vi "子VI-图像预处理.vi"(7 "图像分辨率":T2, 8 "穿透图":T1(plugin-control), 9 "穿透图原始路径":path) -> (1 "穿透图out":T1(plugin-control))   [LabVIEW 2018]
uses:
  <vilib>/vision/NI_Vision_Development_Module.lvlib
panel:
  in  "stop":bool caption="停止"
  in  "图像预处理":bool
  in  "自定义色彩":bool
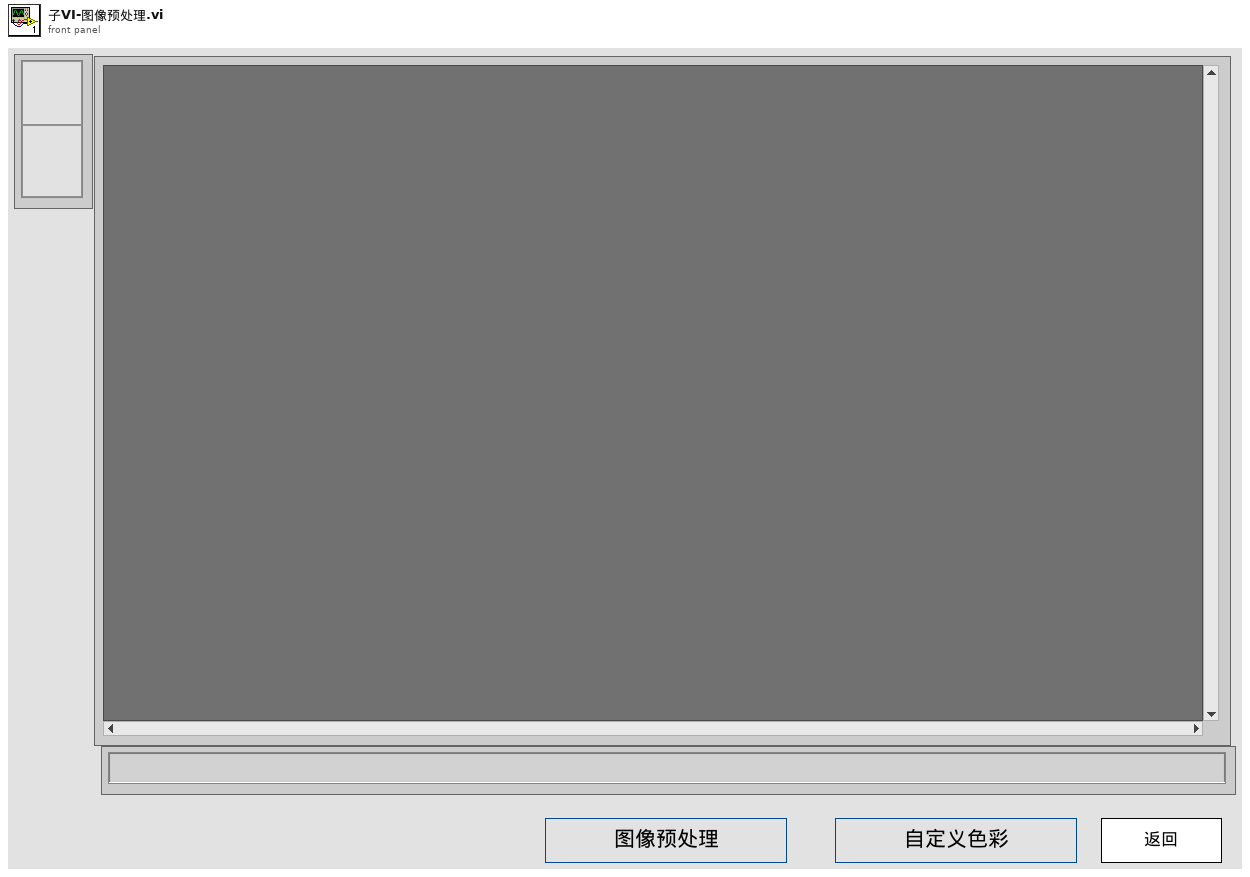
[diagram p1: front panel]
types:
  T1 = typedef "IMAQ Image.ctl" = refnum<image>
  T2 = cluster{"图像X向分辨率（mm/像素）":dbl, "图像Y向分辨率（mm/像素）":dbl}
  T3 = cluster{"Zoom Tool":bool, "Selection Tool":bool, "Pan Tool":bool, "Point Tool":bool, "Line Tool":bool, "Rectangle Tool":bool, "Rotated Rectangle Tool":bool, "Polyline Tool":bool, "Polygon Tool":bool, "Freehand Tool":bool, "Closed Freehand Tool":bool, "Ellipse Tool":bool, "Annulus Tool":bool}
  T4 = enum32{"Linear", "Log", "Exp", "Square", "Square root", "Power X", "Power 1/X"}
  T5 = enum32{"Gray", "Binary", "Gradient", "Rainbow", "Temperature"}
  T6 = enum32{"Invalid", "Standard", "Closed", "Hidden", "Minimized", "Maximized"}
  T7 = typedef "Image Type" = u32
  T8 = cluster{"Red (or Hue) value":u8, "Green (or Sat) value":u8, "Blue (or Light or Val) value":u8}[]
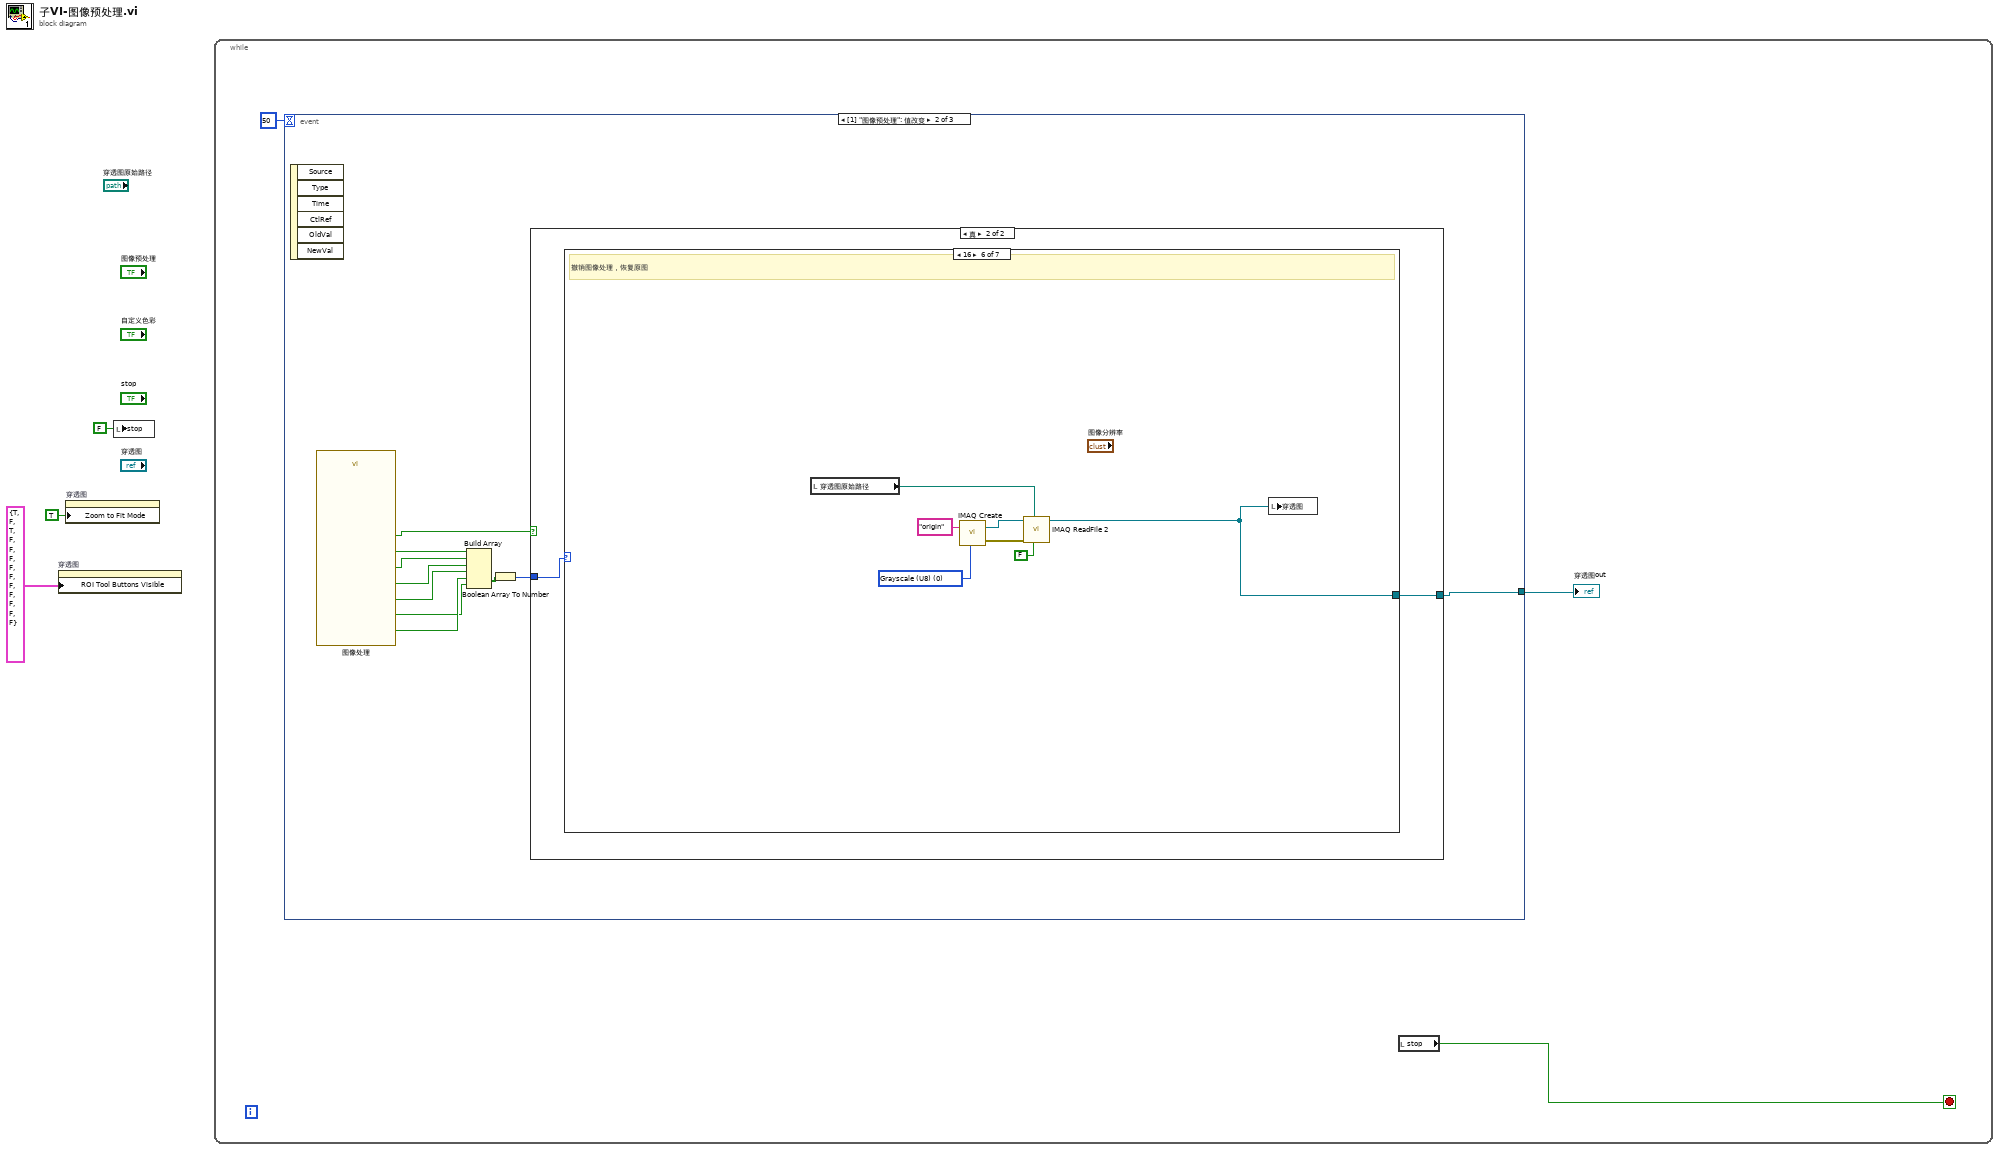
[diagram p0: block diagram]
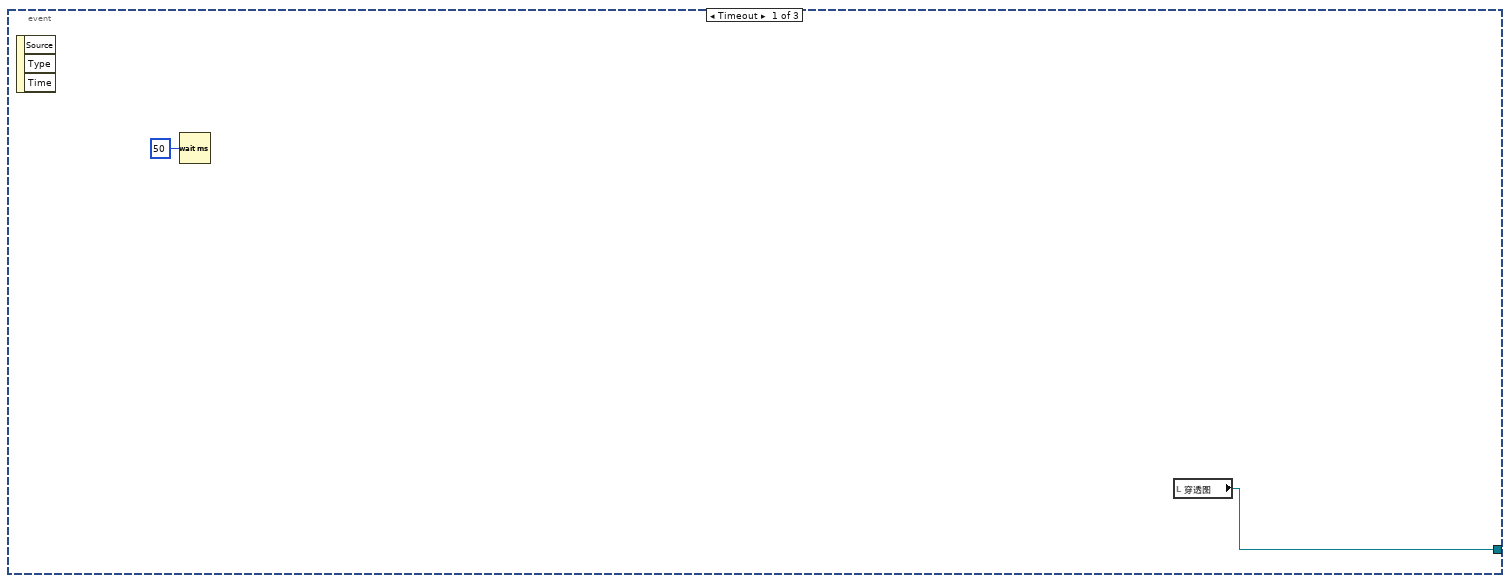
[diagram p2: hidden frame]
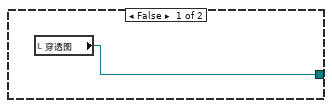
[diagram p3: hidden frame]
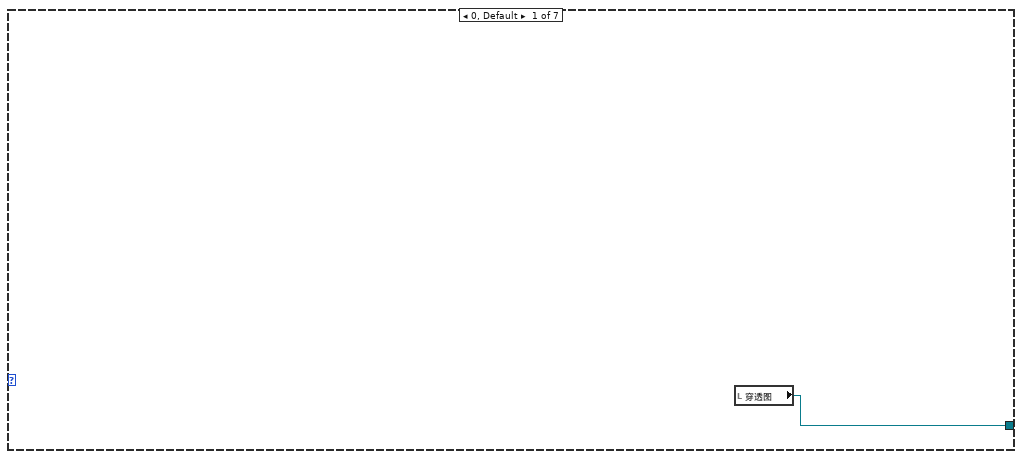
[diagram p4: hidden frame]
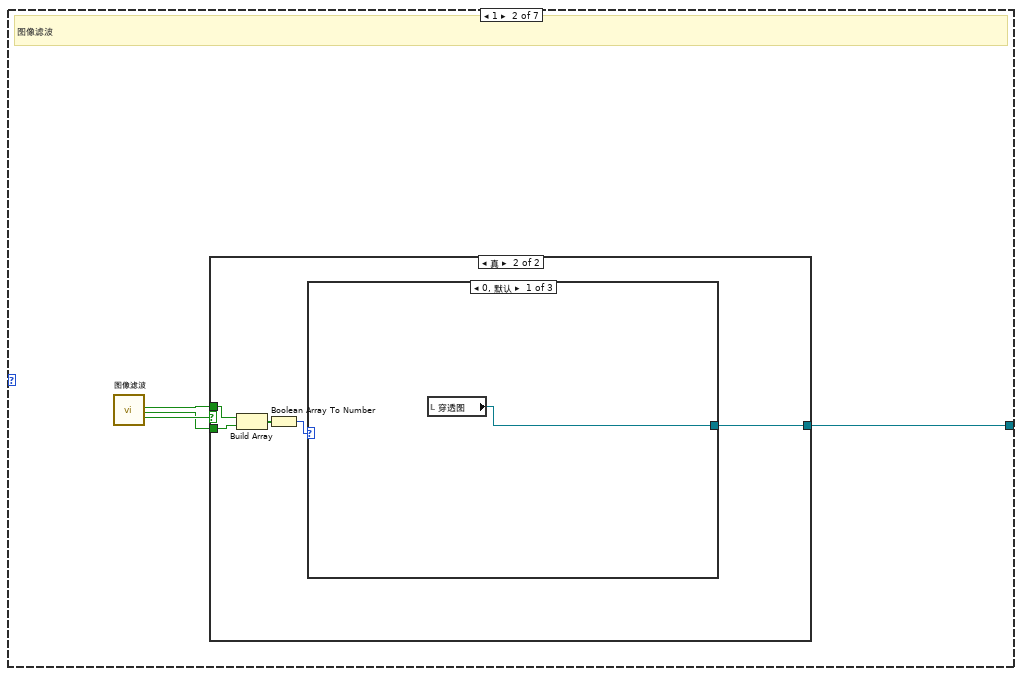
[diagram p5: hidden frame]
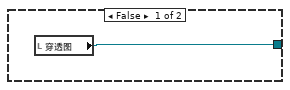
[diagram p6: hidden frame]
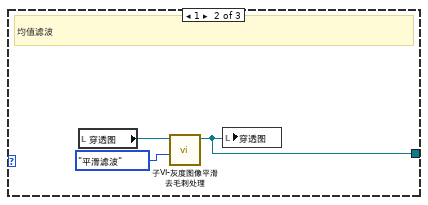
[diagram p7: hidden frame]
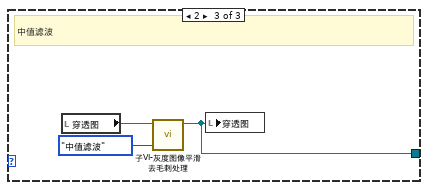
[diagram p8: hidden frame]
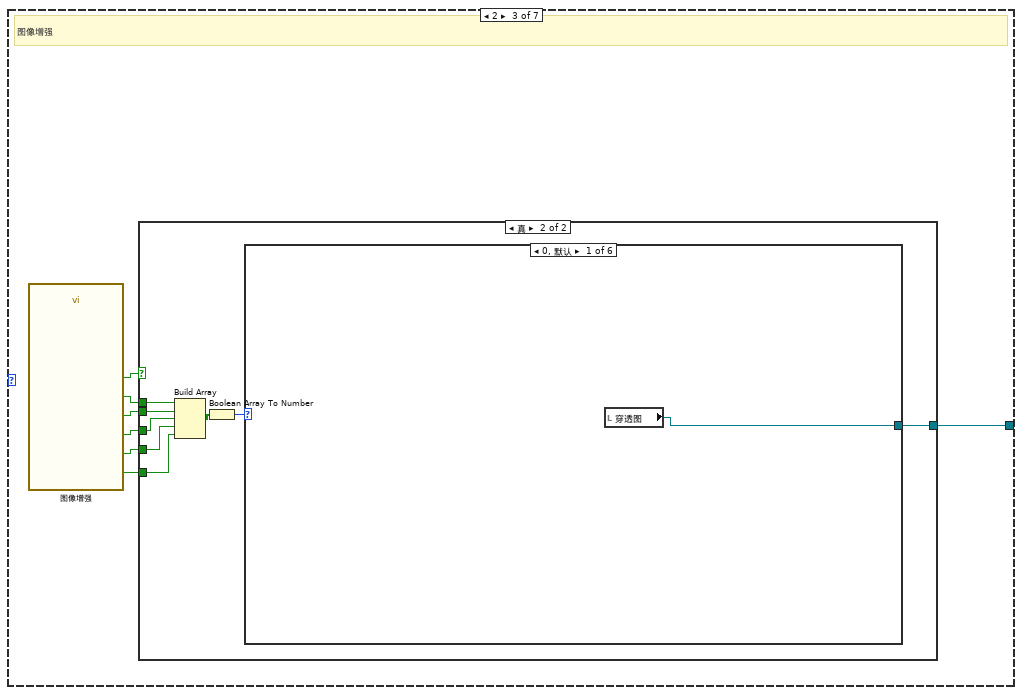
[diagram p9: hidden frame]
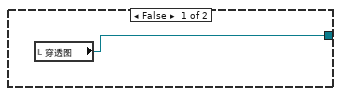
[diagram p10: hidden frame]
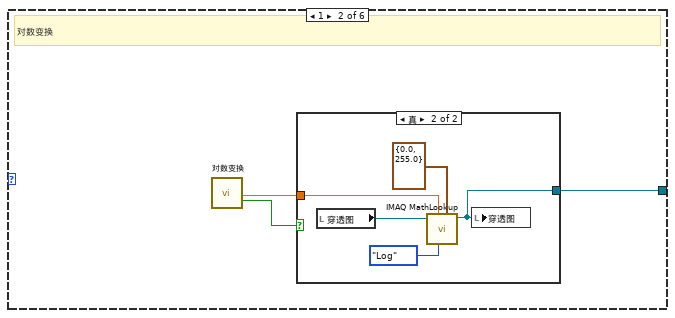
[diagram p11: hidden frame]
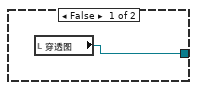
[diagram p12: hidden frame]
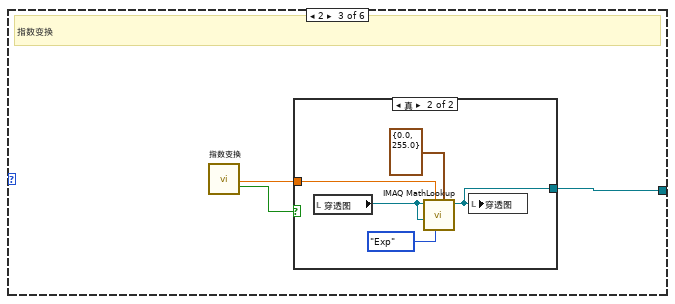
[diagram p13: hidden frame]
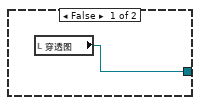
[diagram p14: hidden frame]
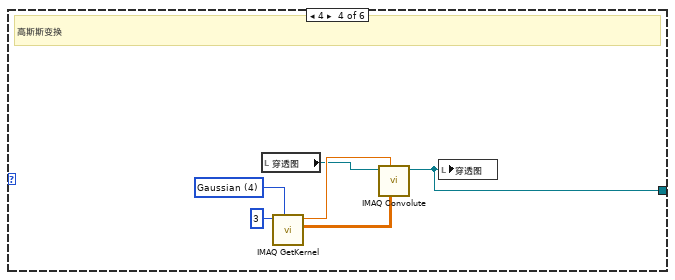
[diagram p15: hidden frame]
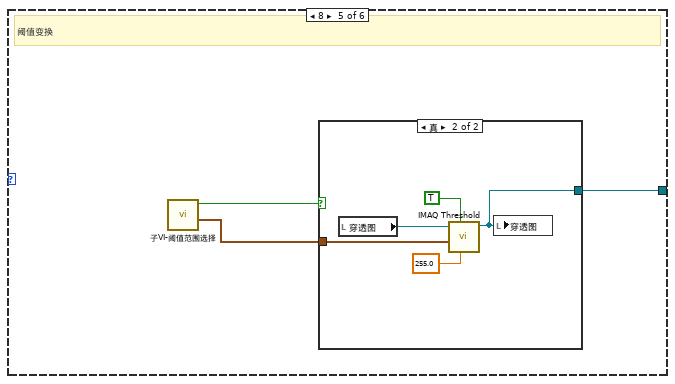
[diagram p16: hidden frame]
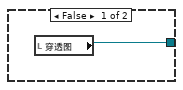
[diagram p17: hidden frame]
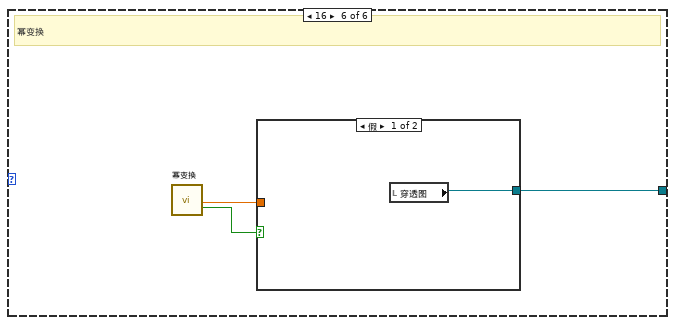
[diagram p18: hidden frame]
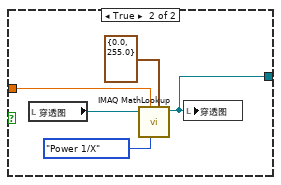
[diagram p19: hidden frame]
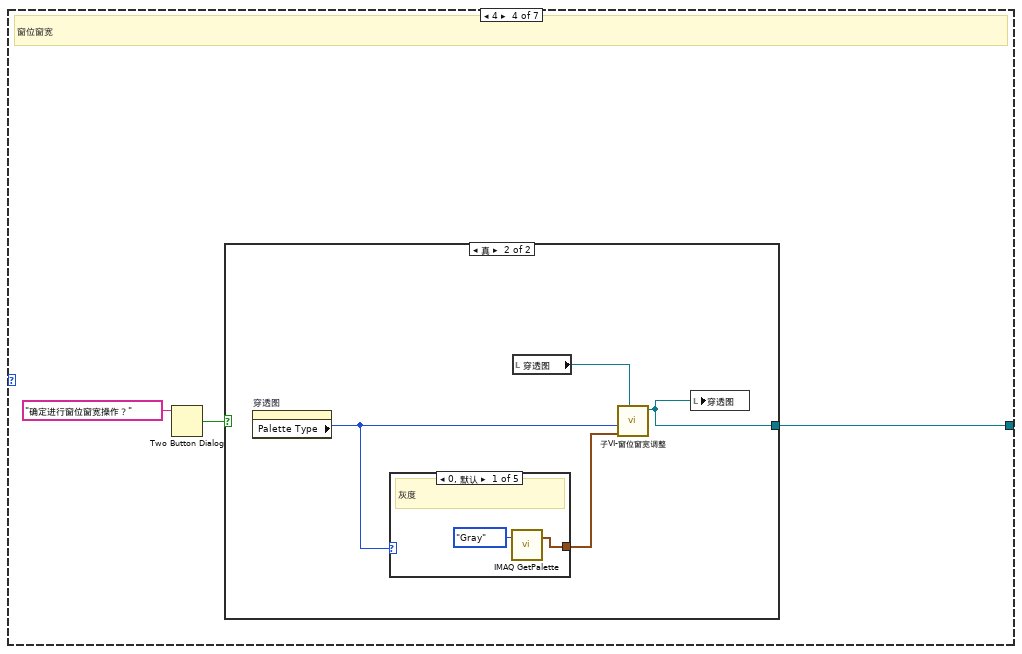
[diagram p20: hidden frame]
diagram:
  n1 = property on="穿透图" class="ImageControl"("ROI Tool Buttons Visible"=T3 {"Zoom Tool"=TRUE, "Selection Tool"=FALSE, "Pan Tool"=TRUE, "Point Tool"=FALSE, "Line Tool"=FALSE, "Rectangle Tool"=FALSE, "Rotated Rectangle Tool"=FALSE, "Polyline Tool"=FALSE, "Polygon Tool"=FALSE, "Freehand Tool"=FALSE, "Closed Freehand Tool"=FALSE, "Ellipse Tool"=FALSE, "Annulus Tool"=FALSE} ("ROI Tool Buttons Visible:All Elements")) -> ()  [unwired: 2 in, 2 out]
  n2 = property on="穿透图" class="ImageControl"("Zoom to Fit Mode"=TRUE) -> ()  [unwired: 2 in, 2 out]
  n3 = local write "stop"(FALSE ("stop")) -> ()
  n4 = while {
    stop <- w6 stop-if-true
    n5 = event shown="[1] \"图像预处理\": 值改变" {
      selector: _ -> [_ _ _]
      dyn-events: _ -> [_ _ _]
      timeout: 50 -> [_ _ _]
      tunnel: [w7 w9 w147] -> w4
      event Timeout {
        n6 = event-data() -> ()  [unwired: 1 in, 3 out]
        n7 = Wait (ms)(milliseconds to wait=u32 50 ("等待时间（毫秒）")) -> ()  [unwired: 1 out]
        n8 = local read "穿透图"() -> (w7:T1)
      }
      event "图像预处理": Value Change {
        n9 = event-data() -> ()  [unwired: 1 in, 6 out]
        n10 = call "图像处理"() -> ("图像反色"=w10:bool, "撤销图像处理"=w13:bool, "线性灰度值测量"=w14:bool, "窗位窗宽"=w17:bool, "图像增强"=w15:bool, "图像滤波"=w18:bool, "确定"=w12:bool)  [unwired: 12 in, 1 out]
        n11 = Build Array(w18, w15, w17, w14, w13, w10) -> (w16:bool[])
        n12 = Boolean Array To Number(Boolean array=w16) -> (number=w11:u32)
        n13 = case shown="真" w12 {
          tunnel: w11 -> [_ w21]
          tunnel: [w19 w20] -> w9
          frame False {
            n14 = local read "穿透图"() -> (w19:T1)
          }
          frame True {
            n15 = case shown="16" w21 {
              tunnel: [w22 w23 w40 w99 w116 w138 w145] -> w20
              frame 0, Default {
                n16 = local read "穿透图"() -> (w22:T1)
              }
              frame 1 {
                # "图像滤波"
                n17 = call "图像滤波"() -> ("均值滤波"=w25:bool, "中值滤波"=w24:bool, "确定"=w26:bool)  [unwired: 16 in, 1 out]
                n18 = case shown="真" w26 {
                  tunnel: w25 -> [_ w31]
                  tunnel: w24 -> [_ w30]
                  tunnel: [w27 w28] -> w23
                  frame False {
                    n19 = local read "穿透图"() -> (w27:T1)
                  }
                  frame True {
                    n20 = Build Array(w31, w30) -> (w32:bool[])
                    n21 = Boolean Array To Number(Boolean array=w32) -> (number=w29:u32)
                    n22 = case shown="0, 默认" w29 {
                      tunnel: [w33 w34 w37] -> w28
                      frame 0, Default {
                        n23 = local read "穿透图"() -> (w33:T1)
                      }
                      frame 1 {
                        # "均值滤波"
                        n24 = local read "穿透图"() -> (w36:T1)
                        n25 = call "子VI-灰度图像平滑去毛刺处理.vi"("滤波方法选择"=enum16{"中值滤波", "平滑滤波"}."平滑滤波", "Image"=w36) -> ("Image Out"=w34:T1)  [unwired: 9 in]
                        n26 = local write "穿透图"(w34) -> ()
                      }
                      frame 2 {
                        # "中值滤波"
                        n27 = local read "穿透图"() -> (w39:T1)
                        n28 = call "子VI-灰度图像平滑去毛刺处理.vi"("滤波方法选择"=enum16{"中值滤波", "平滑滤波"}."中值滤波", "Image"=w39) -> ("Image Out"=w37:T1)  [unwired: 9 in]
                        n29 = local write "穿透图"(w37) -> ()
                      }
                    }
                  }
                }
              }
              frame 2 {
                # "图像增强"
                n30 = call "图像增强"() -> ("幂变换"=w41:bool, "阈值变换"=w42:bool, "高斯变换"=w43:bool, "指数变换"=w44:bool, "对数变换"=w45:bool, "确定"=w46:bool)  [unwired: 13 in, 1 out]
                n31 = case shown="真" w46 {
                  tunnel: w45 -> [_ w53]
                  tunnel: w44 -> [_ w52]
                  tunnel: w43 -> [_ w51]
                  tunnel: w42 -> [_ w50]
                  tunnel: w41 -> [_ w49]
                  tunnel: [w47 w48] -> w40
                  frame False {
                    n32 = local read "穿透图"() -> (w47:T1)
                  }
                  frame True {
                    n33 = Build Array(w53, w52, w51, w50, w49) -> (w55:bool[])
                    n34 = Boolean Array To Number(Boolean array=w55) -> (number=w54:u32)
                    n35 = case shown="0, 默认" w54 {
                      tunnel: [w56 w57 w66 w75 w81 w90] -> w48
                      frame 0, Default {
                        n36 = local read "穿透图"() -> (w56:T1)
                      }
                      frame 1 {
                        # "对数变换"
                        n37 = call "对数变换"() -> ("变换系数K"=w58:dbl, "确定"=w59:bool)  [unwired: 17 in, 1 out]
                        n38 = case shown="真" w59 {
                          tunnel: w58 -> [_ w63]
                          tunnel: [w60 w61] -> w57
                          frame False {
                            n39 = local read "穿透图"() -> (w60:T1)
                          }
                          frame True {
                            n40 = local read "穿透图"() -> (w62:T1)
                            n41 = call "IMAQ MathLookup"("Range"=cluster{"Minimum":sgl, "Maximum":sgl} {"Minimum"=0.0, "Maximum"=255.0}, "Operator"=T4."Log", "X Value"=w63, "Image Src"=w62) -> ("Image Dst Out"=w61:T1)  [unwired: 6 in, 1 out]
                            n42 = local write "穿透图"(w61) -> ()
                          }
                        }
                      }
                      frame 2 {
                        # "指数变换"
                        n43 = call "指数变换"() -> ("变换系数K"=w67:dbl, "确定"=w68:bool)  [unwired: 17 in, 1 out]
                        n44 = case shown="真" w68 {
                          tunnel: w67 -> [_ w71]
                          tunnel: [w69 w70] -> w66
                          frame False {
                            n45 = local read "穿透图"() -> (w69:T1)
                          }
                          frame True {
                            n46 = local read "穿透图"() -> (w74:T1)
                            n47 = call "IMAQ MathLookup"("Range"=cluster{"Minimum":sgl, "Maximum":sgl} {"Minimum"=0.0, "Maximum"=255.0}, "Operator"=T4."Exp", "X Value"=w71, "Image Dst"=w74, "Image Src"=w74) -> ("Image Dst Out"=w70:T1)  [unwired: 5 in, 1 out]
                            n48 = local write "穿透图"(w70) -> ()
                          }
                        }
                      }
                      frame 4 {
                        w80 = u16 4 items=["Gradient"=1, "Laplacian"=2, "Smoothing"=3, "Gaussian"=4] ("Kernel Family")
                        # "高斯斯变换"
                        n49 = local read "穿透图"() -> (w76:T1)
                        n50 = call "IMAQ GetKernel"("Kernel Family"=w80, "Kernel Size (3,5,...)"=3) -> ("Kernel"=w78:sgl[][], "Divider"=w77:sgl)  [unwired: 6 in, 2 out]
                        n51 = call "IMAQ Convolute"("Kernel"=w78, "Divider (kernel sum)"=w77, "Image Src"=w76) -> ("Image Dst Out"=w75:T1)  [unwired: 7 in, 1 out]
                        n52 = local write "穿透图"(w75) -> ()
                      }
                      frame 8 {
                        # "阈值变换"
                        n53 = call "子VI-阈值范围选择.vi"() -> ("阈值范围"=w82:cluster{"Lower value":sgl, "Upper value":sgl}, "确定执行"=w83:bool)  [unwired: 10 in]
                        n54 = case shown="真" w83 {
                          tunnel: w82 -> [_ w88]
                          tunnel: [w84 w85] -> w81
                          frame False {
                            n55 = local read "穿透图"() -> (w84:T1)
                          }
                          frame True {
                            n56 = local read "穿透图"() -> (w86:T1)
                            n57 = call "IMAQ Threshold"("Replace Value"=sgl 255.0, "Keep/Replace Value (Replace)"=TRUE, "Range"=w88, "Image Src"=w86) -> ("Image Dst Out"=w85:T1)  [unwired: 6 in, 1 out]
                            n58 = local write "穿透图"(w85) -> ()
                          }
                        }
                      }
                      frame 16 {
                        # "幂变换"
                        n59 = call "幂变换"() -> ("变换系数K"=w91:dbl, "确定"=w92:bool)  [unwired: 17 in, 1 out]
                        n60 = case shown="假" w92 {
                          tunnel: w91 -> [_ w96]
                          tunnel: [w93 w94] -> w90
                          frame False {
                            n61 = local read "穿透图"() -> (w93:T1)
                          }
                          frame True {
                            n62 = local read "穿透图"() -> (w95:T1)
                            n63 = call "IMAQ MathLookup"("Range"=cluster{"Minimum":sgl, "Maximum":sgl} {"Minimum"=0.0, "Maximum"=255.0}, "Operator"=T4."Power 1/X", "X Value"=w96, "Image Src"=w95) -> ("Image Dst Out"=w94:T1)  [unwired: 6 in, 1 out]
                            n64 = local write "穿透图"(w94) -> ()
                          }
                        }
                      }
                    }
                  }
                }
              }
              frame 4 {
                # "窗位窗宽"
                n65 = Two Button Dialog(message="确定进行窗位窗宽操作？" ("消息")) -> (T button?=w101:bool)  [unwired: 2 in]
                n66 = case shown="真" w101 {
                  tunnel: [w102 w103] -> w99
                  frame False {
                    n67 = local read "穿透图"() -> (w102:T1)
                  }
                  frame True {
                    n68 = property on="穿透图" class="ImageControl"() -> ("Palette Type"=w104:u32)  [unwired: 2 in, 2 out]
                    n69 = case shown="0, 默认" w104 {
                      tunnel: [w107 w109 w111 w113 w115] -> w106
                      frame 0, Default {
                        # "灰度"
                        n70 = call "IMAQ GetPalette"("Palette Number (gray)"=T5."Gray") -> ("Color Palette"=w107:cluster{"Red":u8, "Green":u8, "Blue":u8}[])  [unwired: 4 in, 1 out]
                      }
                      frame 2 {
                        # "梯度"
                        n71 = call "IMAQ GetPalette"("Palette Number (gray)"=T5."Gradient") -> ("Color Palette"=w109:cluster{"Red":u8, "Green":u8, "Blue":u8}[])  [unwired: 4 in, 1 out]
                      }
                      frame 3 {
                        # "彩虹"
                        n72 = call "IMAQ GetPalette"("Palette Number (gray)"=T5."Rainbow") -> ("Color Palette"=w111:cluster{"Red":u8, "Green":u8, "Blue":u8}[])  [unwired: 4 in, 1 out]
                      }
                      frame 4 {
                        # "温度"
                        n73 = call "IMAQ GetPalette"("Palette Number (gray)"=T5."Temperature") -> ("Color Palette"=w113:cluster{"Red":u8, "Green":u8, "Blue":u8}[])  [unwired: 4 in, 1 out]
                      }
                      frame 5 {
                        # "自定义"
                        n74 = property on="穿透图" class="ImageControl"() -> ("User Palette"=w115:cluster{"Red":u8, "Green":u8, "Blue":u8}[])  [unwired: 2 in, 2 out]
                      }
                    }
                    n75 = local read "穿透图"() -> (w105:T1)
                    n76 = call "子VI-窗位窗宽调整.vi"("Image in"=w105, "Palette:User Palette"=w106, "Palette:Palette Type"=w104) -> ("Image out"=w103:T1)  [unwired: 8 in]
                    n77 = local write "穿透图"(w103) -> ()
                  }
                }
              }
              frame 8 {
                # "查看线灰度值曲线，用于精确测量"
                n78 = Current VI's Path() -> (path=w123:path)
                n79 = Open VI Reference(vi path=w123) -> (vi reference=w122:refnum<vi>, error out=w120:errorcluster)  [unwired: 5 in]
                n80 = property class="VI"(reference=w122, error in=w120, "FP.State"=T6."Hidden" ("前面板窗口:状态")) -> (reference out=w121:refnum<vi>, error out=w119:errorcluster)
                n81 = Close Reference(reference=w121, error in (no error)=w119) -> (error out=w117:errorcluster)
                n82 = case shown="无错误" w117 {
                  tunnel: [w124 w137] -> w116
                  frame No Error {
                    n83 = property on="穿透图" class="ImageControl"() -> ("Palette Type"=w125:u32)  [unwired: 2 in, 2 out]
                    n84 = case shown="5" w125 {
                      tunnel: [w128 w130 w132 w134 w136] -> w126
                      frame 0, Default {
                        # "灰度"
                        n85 = call "IMAQ GetPalette"("Palette Number (gray)"=T5."Gray") -> ("Color Palette"=w128:cluster{"Red":u8, "Green":u8, "Blue":u8}[])  [unwired: 4 in, 1 out]
                      }
                      frame 2 {
                        # "梯度"
                        n86 = call "IMAQ GetPalette"("Palette Number (gray)"=T5."Gradient") -> ("Color Palette"=w130:cluster{"Red":u8, "Green":u8, "Blue":u8}[])  [unwired: 4 in, 1 out]
                      }
                      frame 3 {
                        # "彩虹"
                        n87 = call "IMAQ GetPalette"("Palette Number (gray)"=T5."Rainbow") -> ("Color Palette"=w132:cluster{"Red":u8, "Green":u8, "Blue":u8}[])  [unwired: 4 in, 1 out]
                      }
                      frame 4 {
                        # "温度"
                        n88 = call "IMAQ GetPalette"("Palette Number (gray)"=T5."Temperature") -> ("Color Palette"=w134:cluster{"Red":u8, "Green":u8, "Blue":u8}[])  [unwired: 4 in, 1 out]
                      }
                      frame 5 {
                        # "自定义"
                        n89 = property on="穿透图" class="ImageControl"() -> ("User Palette"=w136:cluster{"Red":u8, "Green":u8, "Blue":u8}[])  [unwired: 2 in, 2 out]
                      }
                    }
                    n90 = local read "穿透图"() -> (w124:T1)
                    n91 = local read "图像分辨率"() -> (w127:T2)
                    n92 = call "子VI-线性灰度值曲线查看.vi"("Palette:User Palette"=w126, "图像分辨率"=w127, "Image"=w124) -> ()  [unwired: 9 in]
                  }
                  frame Error {
                    n93 = local read "穿透图"() -> (w137:T1)
                  }
                }
              }
              frame 16 {
                w139 = T7 0 items=["Grayscale (U8)", "Grayscale (I16)", "Grayscale (SGL)", "Complex (CSG)", "RGB (U32)", "HSL (U32)", "RGB (U64)", "Grayscale (U16)"] ("Image Type")
                # "撤销图像处理，恢复原图"
                n94 = local read "穿透图原始路径"() -> (w140:path)
                n95 = call "IMAQ Create"("Image Name"="origin", "Image Type"=w139) -> ("New Image"=w143:T1, "error out"=w144:errorcluster)  [unwired: 3 in]
                n96 = call "IMAQ ReadFile 2"("Use File Path Image Type"=FALSE, "File Path"=w140, "error in (no error)"=w144, "Image"=w143) -> ("Image Out"=w138:T1)  [unwired: 3 in, 4 out]
                n97 = local write "穿透图"(w138) -> ()
              }
              frame 32 {
                # "图像反色 灰度值反转"
                n98 = local read "穿透图"() -> (w146:T1)
                n99 = call "IMAQ Inverse"("Image Src"=w146) -> ("Image Dst Out"=w145:T1)  [unwired: 9 in, 1 out]
                n100 = local write "穿透图"(w145) -> ()
              }
            }
          }
        }
      }
      event "自定义色彩": Value Change {
        n101 = event-data() -> ()  [unwired: 1 in, 6 out]
        n102 = call "调色板"() -> ("自定义显示"=w153:bool, "温度显示"=w152:bool, "彩虹显示"=w151:bool, "梯度显示"=w150:bool, "灰度显示"=w149:bool, "确定"=w148:bool)  [unwired: 13 in, 1 out]
        n103 = Build Array(w149, w150, w151, w152, w153) -> (w154:bool[])
        n104 = case shown="真" w148 {
          tunnel: w154 -> [_ w157]
          frame False {
          }
          frame True {
            n105 = Boolean Array To Number(Boolean array=w157) -> (number=w156:u32)
            n106 = case shown="0, 默认" w156 {
              tunnel: [w158 w159 w160 w161 w162 w164] -> w155
              frame 0, Default {
                w158 = u32 0 items=["Grayscale", "Binary", "Gradient", "Rainbow", "Temperature", "User Defined", "Binary 16 Bit", "Gradient 16 Bit", "Rainbow 16 Bit", "Temperature 16 Bit", "User Defined 16 Bit"] ("Palette:Palette Type")
              }
              frame 1 {
                w159 = u32 0 items=["Grayscale", "Binary", "Gradient", "Rainbow", "Temperature", "User Defined", "Binary 16 Bit", "Gradient 16 Bit", "Rainbow 16 Bit", "Temperature 16 Bit", "User Defined 16 Bit"] ("Palette:Palette Type")
                # "灰度"
              }
              frame 2 {
                w160 = u32 2 items=["Grayscale", "Binary", "Gradient", "Rainbow", "Temperature", "User Defined", "Binary 16 Bit", "Gradient 16 Bit", "Rainbow 16 Bit", "Temperature 16 Bit", "User Defined 16 Bit"] ("Palette:Palette Type")
                # "梯度"
              }
              frame 4 {
                w161 = u32 3 items=["Grayscale", "Binary", "Gradient", "Rainbow", "Temperature", "User Defined", "Binary 16 Bit", "Gradient 16 Bit", "Rainbow 16 Bit", "Temperature 16 Bit", "User Defined 16 Bit"] ("Palette:Palette Type")
                # "彩虹"
              }
              frame 8 {
                w162 = u32 4 items=["Grayscale", "Binary", "Gradient", "Rainbow", "Temperature", "User Defined", "Binary 16 Bit", "Gradient 16 Bit", "Rainbow 16 Bit", "Temperature 16 Bit", "User Defined 16 Bit"] ("Palette:Palette Type")
                # "温度"
              }
              frame 16 {
                w164 = u32 5 items=["Grayscale", "Binary", "Gradient", "Rainbow", "Temperature", "User Defined", "Binary 16 Bit", "Gradient 16 Bit", "Rainbow 16 Bit", "Temperature 16 Bit", "User Defined 16 Bit"] ("Palette:Palette Type")
                # "自定义"
                n107 = call "自定义成像色谱20200214.vi"() -> ("Color palette"=w163:T8)  [unwired: 8 in, 1 out]
                n108 = property on="穿透图" class="ImageControl"("User Palette"=w163) -> ()  [unwired: 2 in, 2 out]
              }
            }
            n109 = property on="穿透图" class="ImageControl"("Palette Type"=w155) -> ()  [unwired: 2 in, 2 out]
          }
        }
        n110 = local read "穿透图"() -> (w147:T1)
      }
    }
    "穿透图out" <- w4
    n111 = local read "stop"() -> (w6:bool)
  }
